vi "set_thermocouple_configuration.vi"(8 "error in (no error)":errorcluster, 10 "Thermocouple type":T1="1", 11 "connection ID":refnum<k5>) -> (0 "error out":errorcluster, 3 "connection ID out":refnum<k5>)   [LabVIEW 2018]
uses:
  typedefs/thermocouple_types.ctl
  typedefs/sensor_types.ctl
panel:
  out "bytes written":i32
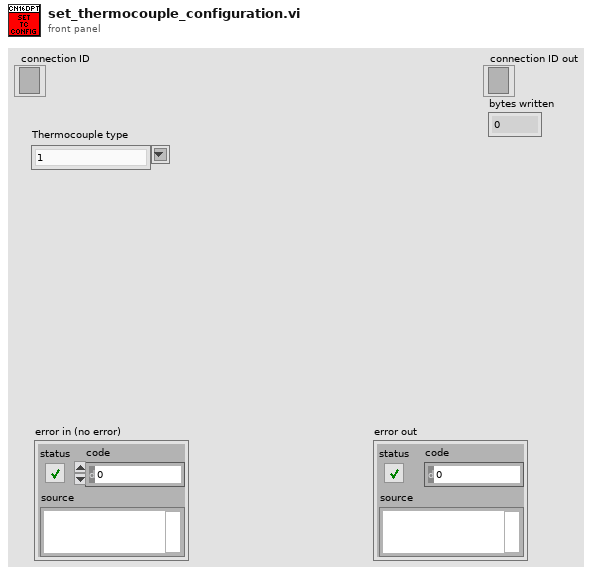
[diagram p1: front panel]
types:
  T1 = typedef "thermocouple_types.ctl" = string
  T2 = typedef "sensor_types.ctl" = string
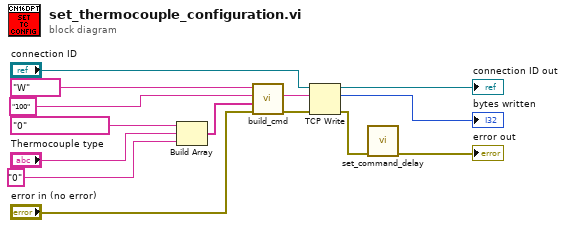
[diagram p0: block diagram]
diagram:
  n1 = Build Array(T2 "0" ("Sensor type"), "Thermocouple type", "0" ("element")) -> (w13:T1[])
  n2 = call "build_cmd.vi"("error in (no error)"="error in (no error)", "Parameter list"=w13, "Command ID"="100", "Command class"="W") -> ("error out"=w10:errorcluster, "Command"=w9:string)  [unwired: 6 in]
  n3 = TCP Write(connection ID="connection ID", data in=w9, error in (no error)=w10) -> (connection ID out=→"connection ID out":refnum<k5>, bytes written=→"bytes written":i32, error out=w3:errorcluster)  [unwired: 1 in]
  n4 = call "set_command_delay.vi"("error in (no error)"=w3) -> ("error out"=→"error out":errorcluster)  [unwired: 10 in]
